vi "uA_daq_Set_Relay_internal_power_on_off_from_baterry.vi"(8 "error in":errorcluster, 10 "Power ON/OFF DUT":enum16{"Power ON DUT", "Power OFF DUT"}(ring), 11 "USB DAQ":tag="Dev4") -> (0 "error out":errorcluster)   [LabVIEW 2017]
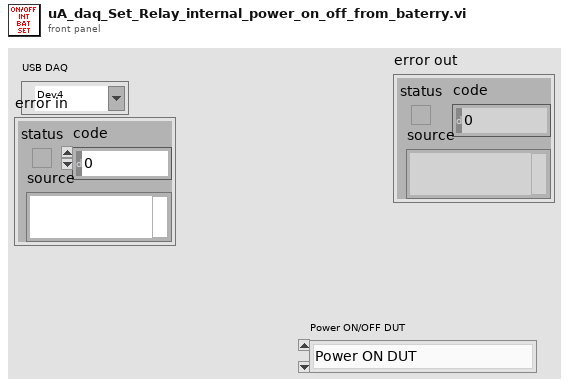
[diagram p1: front panel]
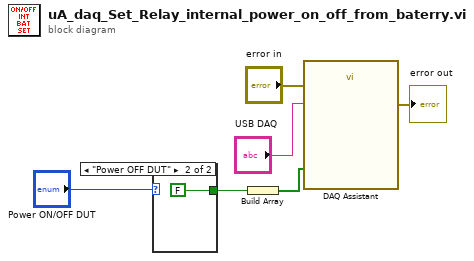
[diagram p0: block diagram]
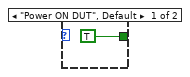
[diagram p2: hidden frame]
diagram:
  n1 = case shown="\"Power OFF DUT\"" "Power ON/OFF DUT" {
    tunnel: [TRUE FALSE] -> w5
    frame "Power ON DUT", Default {
    }
    frame "Power OFF DUT" {
    }
  }
  n2 = Build Array(w5) -> (w4:bool[])
  n3 = call "DAQ Assistant"("data"=w4, "error in"="error in", "device name"="USB DAQ") -> ("error out"=→"error out":errorcluster)  [unwired: 15 in, 1 out]
